vi "CDP1013.vi"() -> ()   [LabVIEW 2020]
uses:
  <vilib>/MakerHub/LINX/Public/Peripherals/Digital/Digital Write N Chans.vi
  <vilib>/MakerHub/LINX/Private/Local IO/LinxDigitalWrite.vi
  <vilib>/MakerHub/LINX/Public/Utilities/Check Channel.vi
  <vilib>/MakerHub/LINX/Public/Utilities/Open Serial.vi
  <vilib>/MakerHub/LINX/Private/Utilties/Generate Error.vi
  <vilib>/MakerHub/LINX/LMH-LINX.lvlib
panel:
  out "Device Name":string
  out "Error Out":errorcluster
  in  "Serial Port":refnum<visa-resource-name>="COM51"
  out "Numeric":i32
  in  "Values":bool[](array[boolean])=[FALSE, FALSE, FALSE, FALSE, FALSE, FALSE, FALSE, FALSE, FALSE, FALSE, FALSE, FALSE, FALSE, FALSE, FALSE, FALSE, FALSE, FALSE, FALSE, FALSE]
  in  "stop":bool
  # "R09 :  DCIR                                   \n\nR10 :  /DCIR\n\nR11 : /CT1  -->ISO+\n\n--dcir/\n\n--dcir\n\nR14 : /CT3 -->ISO-\n\nR02 : LISO-\n\nR01 : LISO+"
  # "NC\n\nBATT\n\n\nVEH\n\n\nAUTO"
  # "CT3\n/CT3"
  # "CT4\n/CT4"
  # "CT5\n/CT5"
  # "CT6\n/CT6"
  # "--Led ISO+\n\n--Led ZEN8\n\n--Led \n\n--Led"
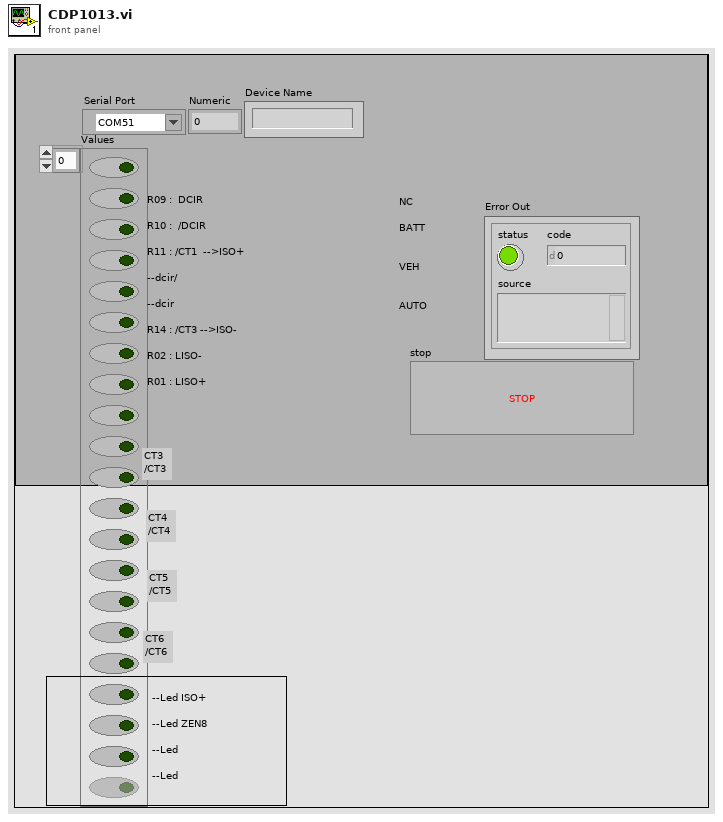
[diagram p1: front panel]
types:
  T1 = typedef "LMH-LINX.lvlib/LINX Ref.ctl" = cluster{"IO":T2, "Interface":T3, "LINX Device Config":T4}
  T2 = typedef "LMH-LINX.lvlib/Platform.ctl" = enum16{"Remote", "Local"}
  T3 = typedef "LMH-LINX.lvlib/Interface.ctl" = enum16{"Serial", "TCP"}
  T4 = typedef "LMH-LINX.lvlib/Device.lvlib/LINX Device Config.ctl" = cluster{"Interface":T3, "COM Port":refnum<visa-resource-name>, "TCP Configuration":T5, "Device Family":u8, "Device ID":u8, "Device Name":string, "TCP Ref":refnum<k5>, "Channels":T6}
  T5 = typedef "LMH-LINX.lvlib/Device.lvlib/TCP Config.ctl" = cluster{"IP Address":string, "Port":u16}
  T6 = typedef "LMH-LINX.lvlib/Channels.ctl" = cluster{"DI":u8[], "DO":u8[], "AI":u8[], "AO":u8[], "PWM":u8[], "QE":u8[], "UART":u8[], "I2C 2":u8[], "SPI":u8[], "CAN":u8[], "Servo":u8[], "AI Ref (V)":dbl, "AI Resolution (Bits)":u8, "AO Ref (V)":dbl, "AO Resolution (Bits)":u8}
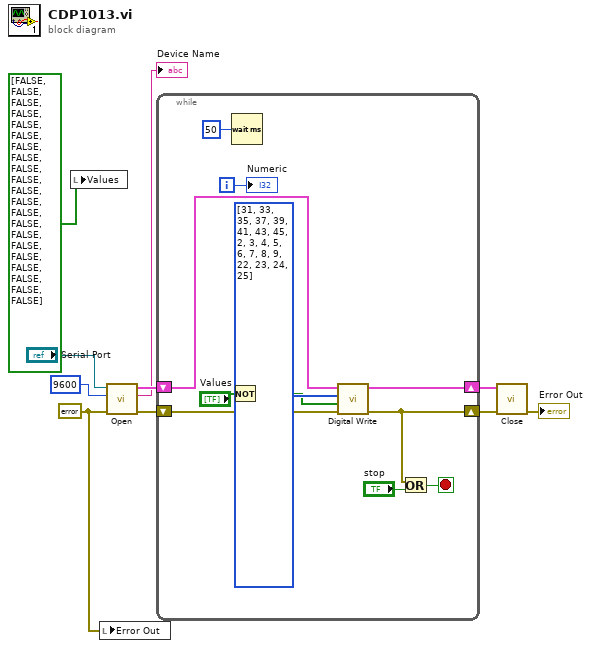
[diagram p0: block diagram]
diagram:
  w3 = errorcluster {"status"=FALSE, "code"=0, "source"=""} ("Error Out")
  n1 = local write "Values"(bool[] [FALSE, FALSE, FALSE, FALSE, FALSE, FALSE, FALSE, FALSE, FALSE, FALSE, FALSE, FALSE, FALSE, FALSE, FALSE, FALSE, FALSE, FALSE, FALSE, FALSE, FALSE] ("Values")) -> ()
  n2 = local write "Error Out"(w3) -> ()
  n3 = call-poly <vilib>:"Open.vi"("Error In"=w3, "Baud Rate Override"=u32 9600, "Serial Port"="Serial Port") -> ("Error Out"=w4:errorcluster, "Device Name"=→"Device Name":string, "LINX Resource"=w7:T1)  [unwired: 6 in]
  n4 = while {
    shift-right: [w15] -> w8
    shift-left: w4 -> [w13]
    shift-right: [w16] -> w6
    shift-left: w7 -> [w14]
    i -> [w20]
    stop <- w17 stop-if-true
    n5 = Not(x="Values") -> (.not. x?=w11:bool[])
    n6 = Wait (ms)(milliseconds to wait=u32 50) -> ()  [unwired: 1 out]
    n7 = call-poly <vilib>:"Digital Write.vi"("Error In"=w13, "Values"=w11, "DO Channels"=u8[] [31, 33, 35, 37, 39, 41, 43, 45, 2, 3, 4, 5, 6, 7, 8, 9, 22, 23, 24, 25], "LINX Resource"=w14) -> ("Error Out"=w15:errorcluster, "LINX Resource"=w16:T1)  [unwired: 6 in]
    n8 = Or(x=w15, y="stop") -> (x .or. y?=w17:bool)
    "Numeric" <- w20
  }
  n9 = call <vilib>:"Close.vi"("Error In"=w8, "LINX Resource"=w6) -> ("Error Out"=→"Error Out":errorcluster)  [unwired: 9 in]
